vi "Configure Burst.vi"(0 "RedPitaya connection in":refnum<k5>, 1 "Number of generated Signals / Burst":i32=-1 min=-1 max=50000, 2 "Number of repeated Bursts":i32=-1 min=-1 max=50000, 3 "Total time of One Burst":i32=-1 min=-1, 4 "Trigger Source":u16(ring) items=["", "EXT_PE", "EXT_NE", "INT", "GATED", "IMM", "IMM BOTH"], 5 "error in":errorcluster, 6 "Channel #":u16(ring) items=["Channel 1"=1, "Channel 2"=2], 12 "timeout ms (2000)":i32=2000) -> (14 "RedPitaya connection out":refnum<k5>, 19 "error out":errorcluster)   [LabVIEW 2010, in "RedPitaya.lvlib"]
doc: "Configures the edge burst trigger mode.\n\nFor parameters <b>Number of generated Signals / Bursts</b> and <b>Number of repeated Bursts</b> you can set the number from 1 to 50000. To set it to infinite, set value to 0."
uses:
  RedPitaya.lvlib
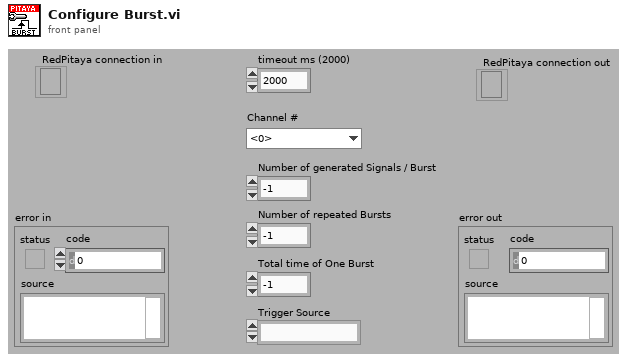
[diagram p1: front panel]
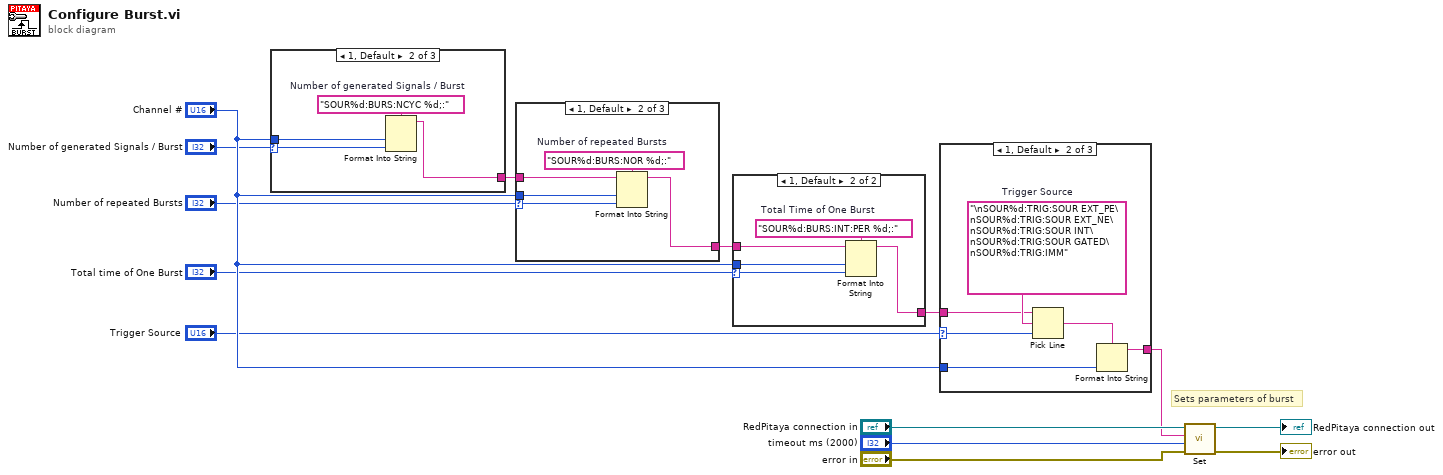
[diagram p0: block diagram]
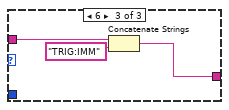
[diagram p3: hidden frame]
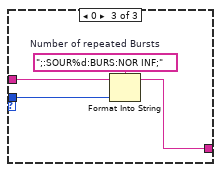
[diagram p6: hidden frame]
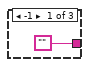
[diagram p7: hidden frame]
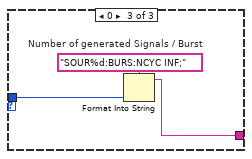
[diagram p8: hidden frame]
diagram:
  # "Sets parameters of burst"
  n1 = case shown="1, Default" "Number of generated Signals / Burst" {
    selector: "Number of generated Signals / Burst" -> [_ w16 _]
    tunnel: ["" w18 w21] -> w10
    tunnel: "Channel #" -> [_ w17 w20]
    frame -1 {
    }
    frame 1, Default {
      w19 = "SOUR%d:BURS:NCYC %d;:"  # Number of generated Signals / Burst
      n2 = Format Into String(format string=w19, w17, w16) -> (resulting string=w18:string)  [unwired: 2 in, 1 out]
    }
    frame 0 {
      w22 = "SOUR%d:BURS:NCYC INF;"  # Number of generated Signals / Burst
      n3 = Format Into String(format string=w22, w20) -> (resulting string=w21:string)  [unwired: 2 in, 1 out]
    }
  }
  n4 = case shown="1, Default" "Number of repeated Bursts" {
    selector: "Number of repeated Bursts" -> [_ w24 _]
    tunnel: w10 -> [w23 w27 w31]
    tunnel: [w23 w26 w30] -> w9
    tunnel: "Channel #" -> [_ w25 w29]
    frame -1 {
    }
    frame 1, Default {
      w28 = "SOUR%d:BURS:NOR %d;:"  # Number of repeated Bursts
      n5 = Format Into String(format string=w28, initial string=w27, w25, w24) -> (resulting string=w26:string)  [unwired: 1 in, 1 out]
    }
    frame 0 {
      w32 = ";:SOUR%d:BURS:NOR INF;"  # Number of repeated Bursts
      n6 = Format Into String(format string=w32, initial string=w31, w29) -> (resulting string=w30:string)  [unwired: 1 in, 1 out]
    }
  }
  n7 = case shown="1, Default" "Total time of One Burst" {
    selector: "Total time of One Burst" -> [_ w34]
    tunnel: w9 -> [w33 w37]
    tunnel: [w33 w36] -> w8
    tunnel: "Channel #" -> [_ w35]
    frame -1 {
    }
    frame 1, Default {
      w38 = "SOUR%d:BURS:INT:PER %d;:"  # Total Time of One Burst
      n8 = Format Into String(format string=w38, initial string=w37, w35, w34) -> (resulting string=w36:string)  [unwired: 1 in, 1 out]
    }
  }
  n9 = case shown="1, Default" "Trigger Source" {
    selector: "Trigger Source" -> [_ w41 _]
    tunnel: w8 -> [w39 w44 w48]
    tunnel: "Channel #" -> [_ w43 _]
    tunnel: [w39 w42 w46] -> w6
    frame 0 {
    }
    frame 1, Default {
      w45 = "\nSOUR%d:TRIG:SOUR EXT_PE\nSOUR%d:TRIG:SOUR EXT_NE\nSOUR%d:TRIG:SOUR INT\nSOUR%d:TRIG:SOUR GATED\nSOUR%d:TRIG:IMM"  # Trigger Source
      n10 = Pick Line(string ("")=w44, multi-line string=w45, line index=w41) -> (output string=w40:string)
      n11 = Format Into String(format string=w40, w43) -> (resulting string=w42:string)  [unwired: 2 in, 1 out]
    }
    frame 6 {
      n12 = Concatenate Strings(w48, "TRIG:IMM" ("string")) -> (w46:string)
    }
  }
  n13 = call "Set.vi"("error in"="error in", "timeout ms (2000)"="timeout ms (2000)", "SCPI Message"=w6, "RedPitaya connection in"="RedPitaya connection in") -> ("error out"=→"error out":errorcluster, "RedPitaya connection out"=→"RedPitaya connection out":refnum<k5>)  [unwired: 5 in, 1 out]
